vi "PID LS Fit Point Array.vi"(0 "response":dbl[](array[numeric]), 1 "TF order":enum16{"1st Order", "2nd Order"}(ring), 5 "length":i32, 9 "noise Band":dbl, 12 "dT":dbl) -> (4 "double integral delta Y":dbl[](array[numeric]), 6 "integral delta Y":dbl[](array[numeric]), 8 "delta Y at t":dbl[](array[numeric]), 10 "time array":dbl[](array[numeric]), 14 "inverse response":bool)   [LabVIEW 2017, in "NI_PID_autopid.lvlib"]
uses:
  <vilib>/addons/control/pid/NI_PID_autopid.lvlib
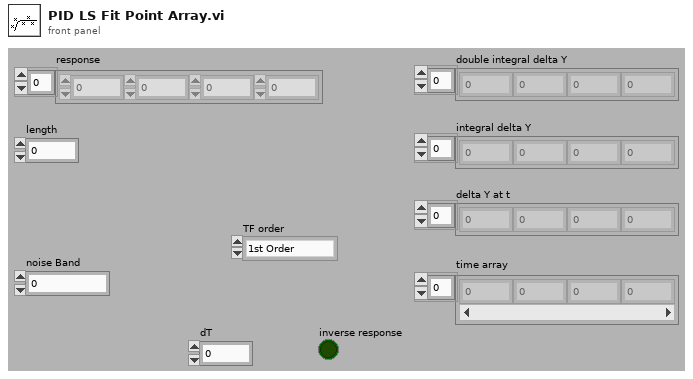
[diagram p1: front panel]
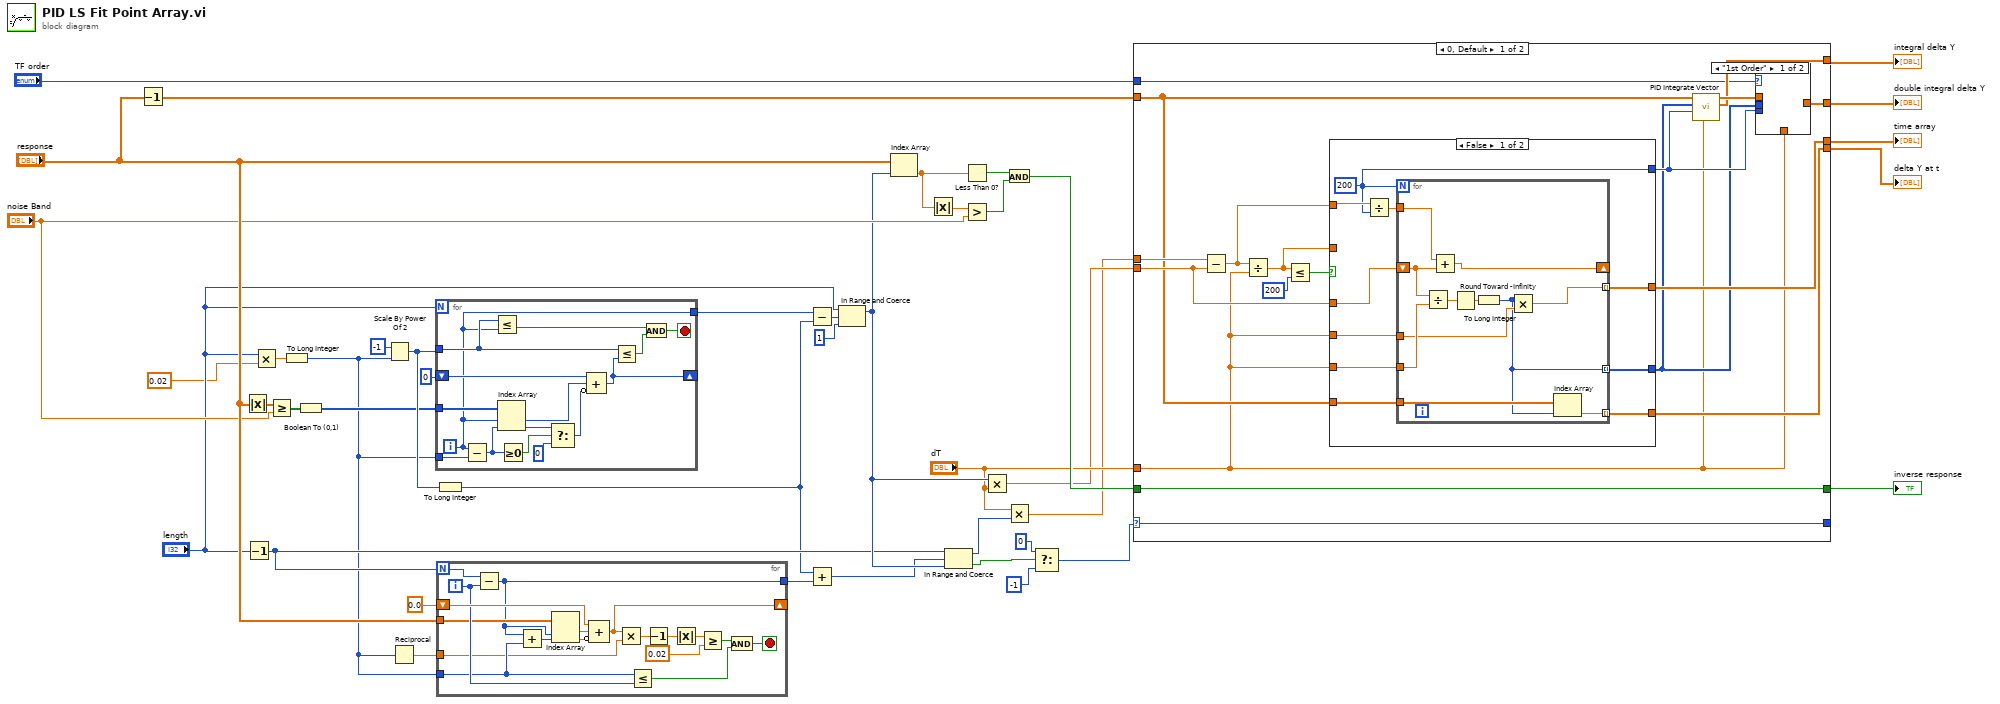
[diagram p0: block diagram]
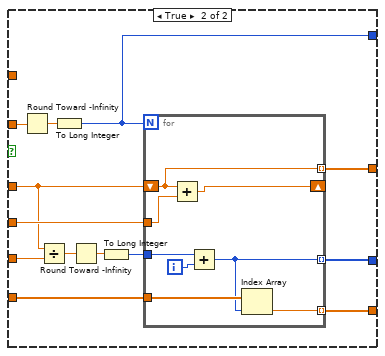
[diagram p2: hidden frame]
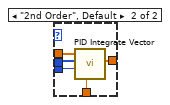
[diagram p3: hidden frame]
diagram:
  n1 = Decrement(x="response") -> (x-1=w33:dbl[])
  n2 = Absolute Value(x="response") -> (abs(x)=w15:dbl[])
  n3 = Decrement(x="length") -> (x-1=w21:i32)
  n4 = Multiply(x="length", y=0.02) -> (x*y=w3:dbl)
  n5 = Greater Or Equal?(x=w15, y="noise Band") -> (x >= y?=w12:bool[])
  n6 = To Long Integer(number=w3) -> (32bit integer=w1:i32)
  n7 = Boolean To (0,1)(Boolean=w12) -> (0, 1=w14:i16[])
  n8 = Scale By Power Of 2(n=-1, x=w1) -> (x*2^n=w27:i32)
  n9 = Reciprocal(x=w1) -> (1/x=w23:dbl)
  n10 = for {
    N: "length" -> [_]
    shift-right: [w54] -> _
    shift-left: i16 0 -> [w57]
    tunnel: w14 -> [w56]
    tunnel: w1 -> [w55]
    tunnel: w27 -> [w53]
    tunnel: [w44] -> w22
    i -> [w44]
    stop <- w50 stop-if-true
    n11 = Subtract(x=w44, y=w55) -> (x-y=w46:i32)
    n12 = Less Or Equal?(x=w53, y=w44) -> (x <= y?=w52:bool)
    n13 = Index Array(array=w56, index #1=w44, index #2=w46) -> (element #1=w43:i16, element #2=w45:i16)
    n14 = Greater Or Equal To 0?(x=w46) -> (x >= 0?=w49:bool)
    n15 = Select(t=w45, s=w49, f=i16 0) -> (s? t:f=w47:i16)
    n16 = Compound Arithmetic op=ADD(w57, w43, invert w47) -> (w54:i16)
    n17 = Less Or Equal?(x=w53, y=w54) -> (x <= y?=w51:bool)
    n18 = And(x=w52, y=w51) -> (x .and. y?=w50:bool)
  }
  n19 = To Long Integer(number=w27) -> (32bit integer=w2:i32)
  n20 = for {
    N: w21 -> [w59]
    shift-right: [w74] -> _
    shift-left: 0.0 -> [w75]
    tunnel: [w61] -> w17
    tunnel: "response" -> [w65]
    tunnel: w1 -> [w60]
    tunnel: w23 -> [w58]
    i -> [w66]
    stop <- w71 stop-if-true
    n21 = Subtract(x=w59, y=w66) -> (x-y=w61:i32)
    n22 = Add(x=w61, y=w60) -> (x+y=w63:i32)
    n23 = Index Array(array=w65, index #1=w61, index #2=w63) -> (element #1=w64:dbl, element #2=w62:dbl)
    n24 = Compound Arithmetic op=ADD(w75, w64, invert w62) -> (w74:dbl)
    n25 = Multiply(x=w74, y=w58) -> (x*y=w70:dbl)
    n26 = Less Or Equal?(x=w60, y=w66) -> (x <= y?=w72:bool)
    n27 = Decrement(x=w70) -> (x-1=w69:dbl)
    n28 = Absolute Value(x=w69) -> (abs(x)=w68:dbl)
    n29 = Greater Or Equal?(x=w68, y=0.02) -> (x >= y?=w73:bool)
    n30 = And(x=w73, y=w72) -> (x .and. y?=w71:bool)
  }
  n31 = Subtract(x=w22, y=w2) -> (x-y=w24:i32)
  n32 = Add(x=w2, y=w17) -> (x+y=w18:i32)
  n33 = In Range and Coerce(upper limit="length", x=w24, lower limit=1) -> (coerced(x)=w26:i32)  [unwired: 1 out]
  n34 = Index Array(array="response", index=w26) -> (element=w28:dbl)
  n35 = Absolute Value(x=w28) -> (abs(x)=w29:dbl)
  n36 = In Range and Coerce(upper limit=w21, x=w18, lower limit=w26) -> (coerced(x)=w19:i32, In Range?=w20:bool)
  n37 = Less Than 0?(x=w28) -> (x < 0?=w30:bool)
  n38 = Greater?(x=w29, y="noise Band") -> (0:w31:bool)
  n39 = Multiply(x=w26, y="dT") -> (x*y=w5:dbl)
  n40 = And(x=w30, y=w31) -> (x .and. y?=w32:bool)
  n41 = Multiply(x="dT", y=w19) -> (x*y=w4:dbl)
  n42 = Select(t=0, s=w20, f=-1) -> (s? t:f=w9:i32)
  n43 = case shown="0, Default" w9 {
    selector: w9 -> [w83 w141]
    tunnel: w4 -> [w93 _]
    tunnel: w5 -> [w92 _]
    tunnel: "dT" -> [w76 _]
    tunnel: [w90 _] -> w41
    tunnel: [w89 _] -> w39
    tunnel: [w88 _] -> w38
    tunnel: "TF order" -> [w87 _]
    tunnel: w33 -> [w85 _]
    tunnel: [w77 _] -> w40
    tunnel: [w83 w141] -> _
    tunnel: w32 -> [w82 _]
    tunnel: [w82 _] -> w34
    frame 0, Default {
      n44 = Subtract(x=w93, y=w92) -> (x-y=w81:dbl)
      n45 = Divide(x=w81, y=w76) -> (x/y=w80:dbl)
      n46 = Less Or Equal?(x=w80, y=200) -> (x <= y?=w79:bool)
      n47 = case shown="False" w79 {
        tunnel: w76 -> [w98 w125]
        tunnel: w92 -> [w101 w121]
        tunnel: w80 -> [_ w126]
        tunnel: [w97 w124] -> w90
        tunnel: w81 -> [w103 _]
        tunnel: w76 -> [w99 w120]
        tunnel: [w100 w118] -> w86
        tunnel: w85 -> [w96 w117]
        tunnel: [w95 w116] -> w77
        tunnel: [w94 w115] -> w84
        frame False {
          w100 = 200
          n48 = Divide(x=w103, y=w100) -> (x/y=w102:dbl)
          n49 = for {
            N: w100 -> [_]
            tunnel: w102 -> [w114]
            shift-right: [w113] -> _
            shift-left: w101 -> [w112]
            tunnel: w99 -> [w111]
            tunnel: w98 -> [w108]
            tunnel: [w107] -> w97 mode=indexing
            tunnel: w96 -> [w106]
            tunnel: [w105] -> w95 mode=indexing
            tunnel: [w104] -> w94 mode=indexing
            n50 = Divide(x=w112, y=w111) -> (x/y=w110:dbl)
            n51 = Add(x=w114, y=w112) -> (x+y=w113:dbl)
            n52 = Round Toward -Infinity(1:w110) -> (0:w109:dbl)
            n53 = To Long Integer(number=w109) -> (32bit integer=w104:i32)
            n54 = Multiply(x=w104, y=w108) -> (x*y=w107:dbl)
            n55 = Index Array(array=w106, index=w104) -> (element=w105:dbl)
          }
        }
        frame True {
          n56 = Round Toward -Infinity(1:w126) -> (0:w127:dbl)
          n57 = Divide(x=w121, y=w120) -> (x/y=w122:dbl)
          n58 = To Long Integer(number=w127) -> (32bit integer=w118:i32)
          n59 = Round Toward -Infinity(1:w122) -> (0:w123:dbl)
          n60 = To Long Integer(number=w123) -> (32bit integer=w119:i32)
          n61 = for {
            N: w118 -> [_]
            tunnel: w125 -> [w135]
            shift-right: [w134] -> _
            shift-left: w121 -> [w133]
            tunnel: [w133] -> w124 mode=indexing
            tunnel: w119 -> [w132]
            tunnel: w117 -> [w130]
            tunnel: [w129] -> w116 mode=indexing
            tunnel: [w128] -> w115 mode=indexing
            i -> [w131]
            n62 = Add(x=w133, y=w135) -> (x+y=w134:dbl)
            n63 = Add(x=w132, y=w131) -> (x+y=w128:i32)
            n64 = Index Array(array=w130, index=w128) -> (element=w129:dbl)
          }
        }
      }
      n65 = call <vilib>:"PID Integrate Vector.vi"("dt"=w76, "Array length"=w86, "Index array"=w84, "Integrate array"=w85) -> ("Timed integration"=w89:dbl[], "Time point results"=w91:dbl[])  [unwired: 6 in]
      n66 = case shown="\"1st Order\"" w87 {
        tunnel: w91 -> [_ w140]
        tunnel: [_ w139] -> w88
        tunnel: w76 -> [_ w138]
        tunnel: w86 -> [_ w137]
        tunnel: w84 -> [_ w136]
        frame "1st Order" {
        }
        frame "2nd Order", Default {
          n67 = call <vilib>:"PID Integrate Vector.vi"("dt"=w138, "Array length"=w137, "Index array"=w136, "Integrate array"=w140) -> ("Timed integration"=w139:dbl[])  [unwired: 6 in, 1 out]
        }
      }
    }
    frame 1 {
    }
  }
  "delta Y at t" <- w40
  "integral delta Y" <- w39
  "double integral delta Y" <- w38
  "time array" <- w41
  "inverse response" <- w34
